vi "class_data.vi"() -> ()   [LabVIEW 2010, in "FPGAWrapperMH120124FrameScan_PXI7813R.lvclass"]
uses:
  FPGAWrapperMH120124FrameScan_PXI7813R.lvclass
  settings_cluster_framescan.ctl
  common_typedefs/channels_cluster.ctl
  fpgaVIsAndControls/DDS_board_init_cluster.ctl
  fpgaVIsAndControls/gate_cluster.ctl
  common_typedefs/gate_parameters_cluster.ctl
  configuration_cluster_framescan.ctl
panel:
  in  "# of callers":i32
  out "ready for initialise?":bool=TRUE
  out "allowed to initialise?":bool=TRUE
  out "configuration writer":refnum<k21>
  out "command writer":refnum<k21>
  out "settings writer":refnum<k21>
  out "data reader 3":refnum<k21>
  out "data reader 2":refnum<k21>
  out "data reader 1":refnum<k21>
  # "FSK"
  # "Ramped"
  # "FSK"
  # "Chirp Modus"
  # "Unramped"
  # "BPSK"
  # "Single Tone"
  # "FSK"
  # "Ramped"
  # "FSK"
  # "Chirp Modus"
  # "Unramped"
  # "BPSK"
  # "Single Tone"
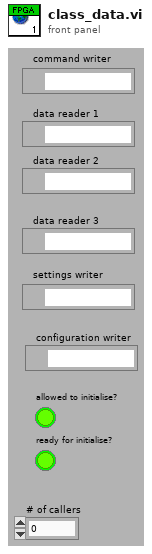
[diagram p1: front panel]
diagram:
